vi "Transform3d_Times.vi"(9 "Scalar":dbl, 11 "in Transform3d":T1={"TRANSLATION3D"={"X"=0.0, "Y"=0.0, "Z"=0.0}, "ROTATION3D"={"Q_quaternion"={"R"=1.0, "V"=[0.0, 0.0, 0.0]}}, "XF"=FALSE} {"TRANSLATION3D"."Z" format="%14.3f"; "TRANSLATION3D"."Y" format="%14.3f"; "TRANSLATION3D"."X" format="%14.3f"}) -> (3 "Transform3d":T1={"TRANSLATION3D"={"X"=0.0, "Y"=0.0, "Z"=0.0}, "ROTATION3D"={"Q_quaternion"={"R"=1.0, "V"=[0.0, 0.0, 0.0]}}, "XF"=FALSE} {"TRANSLATION3D"."Z" format="%14.3f"; "TRANSLATION3D"."Y" format="%14.3f"; "TRANSLATION3D"."X" format="%14.3f"})   [LabVIEW 2019, in "Trajectory_Library.lvlib"]
doc: "Scales the transform3d by the scalar.\n\nParameters:\n - IN TRANSFORM3d -- This TRANSFORM data structure\n - SCALAR -- The scalar value to multiply the transform by\n\nResults:\n - OUT TRANSFORM3d -- The multiplied transform data structure"
uses:
  Trajectory_Library.lvlib
  TypeDef/TRANSLATION3D.ctl
  TypeDef/QUATERNION.ctl
  TypeDef/ROTATION3D.ctl
  TypeDef/TRANSFORM3D.ctl
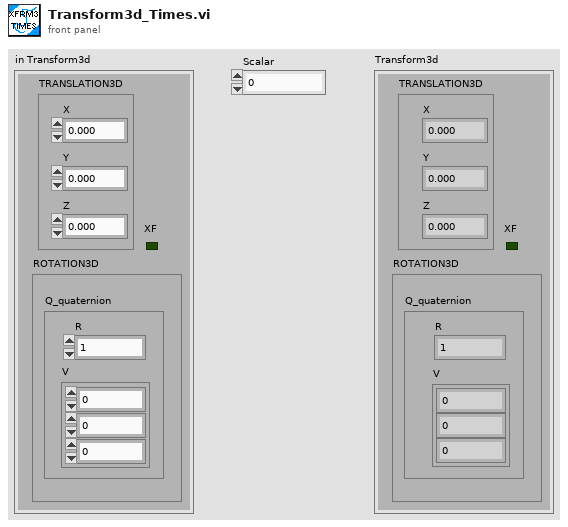
[diagram p1: front panel]
types:
  T1 = typedef "Trajectory_Library.lvlib/TRANSFORM3D.ctl" = cluster{"TRANSLATION3D":T2, "ROTATION3D":T3, "XF":bool}
  T2 = typedef "Trajectory_Library.lvlib/TRANSLATION3D.ctl" = cluster{"X":dbl, "Y":dbl, "Z":dbl}
  T3 = typedef "Trajectory_Library.lvlib/ROTATION3D.ctl" = cluster{"Q_quaternion":T4}
  T4 = typedef "Trajectory_Library.lvlib/QUATERNION.ctl" = cluster{"R":dbl, "V":dbl[]}
  T5 = typedef "WPILib_Math.lvlib/TRANSLATION3D.ctl" = cluster{"X":dbl, "Y":dbl, "Z":dbl}
  T6 = typedef "WPILib_Math.lvlib/ROTATION3D.ctl" = cluster{"Q_quaternion":T7}
  T7 = typedef "WPILib_Math.lvlib/QUATERNION.ctl" = cluster{"R":dbl, "V":dbl[]}
  T8 = typedef "WPILib_Math.lvlib/TRANSFORM3D.ctl" = cluster{"TRANSLATION3D":T5, "ROTATION3D":T6, "XF":bool}
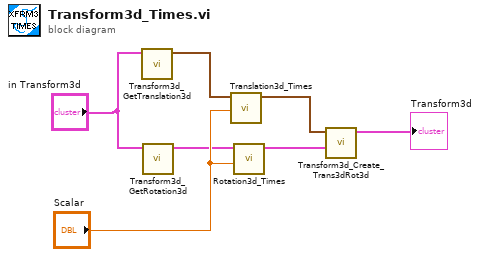
[diagram p0: block diagram]
diagram:
  n1 = call "Transform3d_GetTranslation3d.vi"("in Transform3d"="in Transform3d") -> ("Translation3d"=w2:T2)  [unwired: 10 in]
  n2 = call "Transform3d_GetRotation3d.vi"("in Transform3d"="in Transform3d") -> ("Rotation3d"=w1:T3)  [unwired: 10 in]
  n3 = call "Translation3d_Times.vi"("Scalar"="Scalar", "In Translation3d"=w2) -> ("Out Translation3d"=w3:T5)  [unwired: 9 in]
  n4 = call "Rotation3d_Times.vi"("Scalar"="Scalar", "in Rotation3d"=w1) -> ("out Rotation3d"=w4:T6)  [unwired: 9 in]
  n5 = call "Transform3d_Create_Trans3dRot3d.vi"("Rotation3d"=w4, "Translation3d"=w3) -> ("Transform3d"=→"Transform3d":T8)  [unwired: 9 in]
